vi "BotSpeak_IPAddr.vi"(4 "Bot Settings":T1) -> (0 "response":string="Test", 1 "Bot Settings 2":T1)   [LabVIEW 2012]
doc: "Returns the IP address of the associated RIO as \"response\"."
uses:
  <userlib>/BotSpeak/VIs/Direct/BotSpeak_Control.ctl
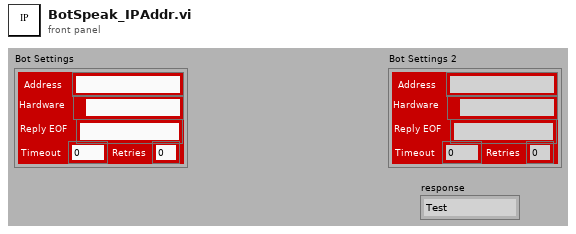
[diagram p1: front panel]
types:
  T1 = typedef "BotSpeak_Control.ctl" = cluster{"Address":string, "Reply EOF":string, "Hardware":path, "Retries":i8, "Timeout":i32}
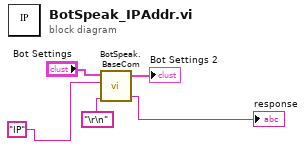
[diagram p0: block diagram]
diagram:
  n1 = call <userlib>:"BotSpeak.BaseCom.vi"("Termination"="\r\n", "command"="IP", "Bot Settings in"="Bot Settings") -> ("response"=→"response":string, "Bot Settings out"=→"Bot Settings 2":T1)  [unwired: 2 in]
